vi "CreatePrivateEvents.vi"(8 "error in (no error)":errorcluster, 11 "Lockin.DAQ":refnum<class "Instrument.DAQ.lvclass">) -> (0 "error out":errorcluster, 3 "Lockin.DAQ out":refnum<class "Instrument.DAQ.lvclass">)   [LabVIEW 2019, in "Instrument.Lockin.lvlib" / "Instrument.DAQ.lvclass"]
doc: "---------------------------------------------------------------\nJKI State Machine Objects™\nhttp://jki.net/state-machine-objects/\nCopyright (C) 2005-2015, JKI <info@jki.net>\nALL RIGHTS RESERVEDJKI State Machine Objects (SMO) 1.0.0.4\nJKI - JKI\nCopyright (c) 2015, JKI"
uses:
  Instrument.DAQ.lvclass
  Typedefs/PrivateEvents--DAQ.setAOconfig.ctl
  Typedefs/DAQ.Config.AO--Cluster--Array.ctl
  Typedefs/DAQ.Config.AO--Cluster.ctl
  Typedefs/DAQ.Config.AO.Range--enum.ctl
  Typedefs/DAQ.Type--enum.ctl
  Typedefs/PrivateEvents--DAQ.setAIconfig.ctl
  Typedefs/DAQ.Config.AI--Cluster--Array.ctl
  Typedefs/DAQ.Config.AI--Cluster.ctl
  Typedefs/DAQ.Config.AI.Coupling--enum.ctl
  Typedefs/DAQ.Config.AI.Range--enum.ctl
  Typedefs/Simulation Mode--enum.ctl
  Typedefs/PrivateEvents--DAQ.setAO.ctl
  Typedefs/AO.Channel--Cluster--Array.ctl
  Typedefs/AO.Channel--Cluster.ctl
  Typedefs/AO.Channel.Function--Enum.ctl
  Typedefs/PrivateEvents--DAQ.setREF.ctl
  Typedefs/REF.Channel--Cluster--Array.ctl
  Typedefs/REF.Channel--Cluster.ctl
  Typedefs/PrivateEvents--DAQ.setSampling.ctl
  Typedefs/DAQ.Sampling--Cluster.ctl
  Typedefs/DAQ.Sampling.Sampling--Cluster.ctl
  Typedefs/DAQ.Sampling.Fs Mode--enum.ctl
  Typedefs/PrivateEvents--DAQ.setState.ctl
  Typedefs/Set State-enum.ctl
  Typedefs/PrivateEvents--DAQ.setInputGain.ctl
  Typedefs/PrivateEvents--DAQ.setSweep.ctl
  Typedefs/Sweep.Configuration--Cluster.ctl
  Typedefs/Sweep.Channel--Cluster--Array.ctl
  Typedefs/Sweep.Channel--Cluster.ctl
  Typedefs/Sweep.Pattern--Enum.ctl
  Typedefs/PrivateEvents--DAQ.measureOffset.ctl
  Typedefs/PrivateEvents--DAQ.zeroOffset.ctl
  Typedefs/PrivateEvents--DAQ.setPreFilter.ctl
  Typedefs/Configuration.Prefilter--Cluster.ctl
  Typedefs/PrivateEvents--DAQ.autoConfigureDAQ.ctl
  Typedefs/PrivateEvents--DAQ.setCalibration.ctl
  Typedefs/PrivateEvents--DAQ.setOutputGain.ctl
  Typedefs/PrivateEvents--DAQ.setAI.ctl
  Typedefs/AI.Channel--Cluster--Array.ctl
  Typedefs/AI.Channel--Cluster.ctl
  Typedefs/PrivateEvents--DAQ.zeroPhase.ctl
  Typedefs/PrivateEvents--DAQ.setAmplitudeLimit.ctl
  Typedefs/Configuration.AmplitudeLimit--Cluster.ctl
  Typedefs/PrivateEvents--DAQ.setLinkFrequencies.ctl
  Typedefs/Configuration.LinkFrequencies--Cluster.ctl
  Typedefs/PrivateEvents--DAQ.showUI.ctl
  Typedefs/PrivateEvents--DAQ.setInputOffset.ctl
  Instrument.DAQ.lvclass/Instrument.DAQ.ctl
  <vilib>/JKI/JKI SMO/SMO/SMO.lvclass
  Typedefs/Configuration.DCLimit--Cluster.ctl
  Typedefs/PrivateEvents--DAQ.setDCLimit.ctl
panel:
  # "For instructions on how to use the JKI State Machine Objects, examples and video tutorials, visit:\nhttp://jki.net/state-machine-objects/\n\nJKI State Machine Objects™\nhttp://jki.net/state-machine-objects/\nCopyright (C) 2005-2015, JKI <info@jki.net>\nALL RIGHTS RESERVED"
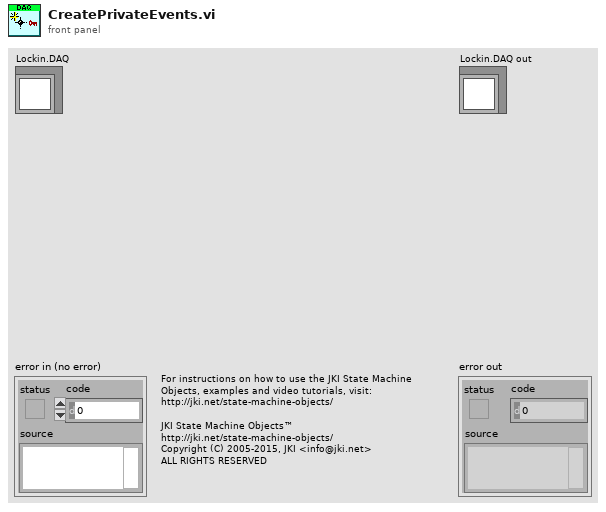
[diagram p1: front panel]
types:
  T1 = typedef "Instrument.Lockin.lvlib/Instrument.DAQ.lvclass/PrivateEvents--DAQ.setDCLimit.ctl" = cluster{"DC Limit":T2}
  T2 = typedef "Instrument.Lockin.lvlib/Instrument.DAQ.lvclass/Configuration.DCLimit--Cluster.ctl" = cluster{"Limit?":bool, "Limit (V)":dbl}
  T3 = typedef "Instrument.Lockin.lvlib/Instrument.DAQ.lvclass/PrivateEvents--DAQ.setInputOffset.ctl" = cluster{"Input Offset":dbl[]}
  T4 = typedef "Instrument.Lockin.lvlib/Instrument.DAQ.lvclass/PrivateEvents--DAQ.showUI.ctl" = bool
  T5 = typedef "Instrument.Lockin.lvlib/Instrument.DAQ.lvclass/PrivateEvents--DAQ.setLinkFrequencies.ctl" = cluster{"Link Frequencies":T6}
  T6 = typedef "Instrument.Lockin.lvlib/Instrument.DAQ.lvclass/Configuration.LinkFrequencies--Cluster.ctl" = cluster{"Link?":bool, "Frequency (Hz)":dbl}
  T7 = typedef "Instrument.Lockin.lvlib/Instrument.DAQ.lvclass/PrivateEvents--DAQ.setAmplitudeLimit.ctl" = cluster{"Amplitude Limit ":T8}
  T8 = typedef "Instrument.Lockin.lvlib/Instrument.DAQ.lvclass/Configuration.AmplitudeLimit--Cluster.ctl" = cluster{"Limit?":bool, "Limit (V)":dbl}
  T9 = typedef "Instrument.Lockin.lvlib/Instrument.DAQ.lvclass/PrivateEvents--DAQ.zeroPhase.ctl" = bool
  T10 = typedef "Instrument.Lockin.lvlib/Instrument.DAQ.lvclass/PrivateEvents--DAQ.setAI.ctl" = cluster{"AI Channels":T11}
  T11 = typedef "Instrument.Lockin.lvlib/Instrument.DAQ.lvclass/AI.Channel--Cluster--Array.ctl" = T12[]
  T12 = typedef "Instrument.Lockin.lvlib/Instrument.DAQ.lvclass/AI.Channel--Cluster.ctl" = cluster{"Enable?":bool, "Channel":i32, "References":i32[]}
  T13 = typedef "Instrument.Lockin.lvlib/Instrument.DAQ.lvclass/PrivateEvents--DAQ.setOutputGain.ctl" = cluster{"Output Gain":dbl[]}
  T14 = typedef "Instrument.Lockin.lvlib/Instrument.DAQ.lvclass/PrivateEvents--DAQ.setCalibration.ctl" = enum16{"Check", "Calibrate"}
  T15 = typedef "Instrument.Lockin.lvlib/Instrument.DAQ.lvclass/PrivateEvents--DAQ.autoConfigureDAQ.ctl" = bool
  T16 = typedef "Instrument.Lockin.lvlib/Instrument.DAQ.lvclass/PrivateEvents--DAQ.setPreFilter.ctl" = cluster{"PreFilter":T17}
  T17 = typedef "Instrument.Lockin.lvlib/Instrument.DAQ.lvclass/Configuration.Prefilter--Cluster.ctl" = cluster{"60 Hz":bool, "Low Pass":bool, "Low Pass Cutoff (Hz)":dbl}
  T18 = typedef "Instrument.Lockin.lvlib/Instrument.DAQ.lvclass/PrivateEvents--DAQ.zeroOffset.ctl" = bool
  T19 = typedef "Instrument.Lockin.lvlib/Instrument.DAQ.lvclass/PrivateEvents--DAQ.measureOffset.ctl" = bool
  T20 = typedef "Instrument.Lockin.lvlib/Instrument.DAQ.lvclass/PrivateEvents--DAQ.setSweep.ctl" = cluster{"setSweep":T21}
  T21 = typedef "Instrument.Lockin.lvlib/Instrument.DAQ.lvclass/Sweep.Configuration--Cluster.ctl" = cluster{"Sweep Time (s)":dbl, "Initial Wait (s)":dbl, "Return to Start":bool, "Channels":T22}
  T22 = typedef "Instrument.Lockin.lvlib/Instrument.DAQ.lvclass/Sweep.Channel--Cluster--Array.ctl" = T23[]
  T23 = typedef "Instrument.Lockin.lvlib/Instrument.DAQ.lvclass/Sweep.Channel--Cluster.ctl" = cluster{"Enable?":bool, "Channel":u16, "Start":dbl, "End":dbl, "Pattern":T24, "Table":dbl[]}
  T24 = typedef "Instrument.Lockin.lvlib/Instrument.DAQ.lvclass/Sweep.Pattern--Enum.ctl" = enum16{"Ramp /", "Ramp /\\", "Smooth Ramp _/", "Smooth Ramp _/\\_", "Table"}
  T25 = typedef "Instrument.Lockin.lvlib/Instrument.DAQ.lvclass/PrivateEvents--DAQ.setInputGain.ctl" = cluster{"Input Gain":dbl[]}
  T26 = typedef "Instrument.Lockin.lvlib/Instrument.DAQ.lvclass/PrivateEvents--DAQ.setState.ctl" = cluster{"setState":T27}
  T27 = typedef "Instrument.Lockin.lvlib/Instrument.DAQ.lvclass/Set State-enum.ctl" = enum16{"start", "stop", "reset", "start sweep", "stop sweep"}
  T28 = typedef "Instrument.Lockin.lvlib/Instrument.DAQ.lvclass/PrivateEvents--DAQ.setSampling.ctl" = cluster{"Sampling":T29}
  T29 = typedef "Instrument.Lockin.lvlib/Instrument.DAQ.lvclass/DAQ.Sampling--Cluster.ctl" = cluster{"Sampling":T30, "sample mode":i32, "Fs Mode":T31, "Fs Multiplier":dbl, "Refresh Rate (Hz)":dbl, "Decimation.PreDSP":i32, "Decimation.PostDSP":i32, "Fs.Output":dbl}
  T30 = typedef "Instrument.Lockin.lvlib/Instrument.DAQ.lvclass/DAQ.Sampling.Sampling--Cluster.ctl" = cluster{"Fs":dbl, "#s":i32}
  T31 = typedef "Instrument.Lockin.lvlib/Instrument.DAQ.lvclass/DAQ.Sampling.Fs Mode--enum.ctl" = enum16{"Manual", "Auto Fs", "Max Fs"}
  T32 = typedef "Instrument.Lockin.lvlib/Instrument.DAQ.lvclass/PrivateEvents--DAQ.setREF.ctl" = cluster{"REF Channels":T33}
  T33 = typedef "Instrument.Lockin.lvlib/Instrument.DAQ.lvclass/REF.Channel--Cluster--Array.ctl" = T34[]
  T34 = typedef "Instrument.Lockin.lvlib/Instrument.DAQ.lvclass/REF.Channel--Cluster.ctl" = cluster{"Enable?":bool, "Channel":i32, "Frequency":dbl, "Phase":dbl, "TC":dbl, "Roll-Off":i32}
  T35 = typedef "Instrument.Lockin.lvlib/Instrument.DAQ.lvclass/PrivateEvents--DAQ.setAO.ctl" = cluster{"AO Channels":T36}
  T36 = typedef "Instrument.Lockin.lvlib/Instrument.DAQ.lvclass/AO.Channel--Cluster--Array.ctl" = T37[]
  T37 = typedef "Instrument.Lockin.lvlib/Instrument.DAQ.lvclass/AO.Channel--Cluster.ctl" = cluster{"Enable?":bool, "Channel":i32, "Amplitude":dbl, "Offset":dbl, "Frequency":dbl, "Phase":dbl, "Function":T38, "Sweeping?":bool}
  T38 = typedef "Instrument.Lockin.lvlib/Instrument.DAQ.lvclass/AO.Channel.Function--Enum.ctl" = enum16{"Sine", "Triangle", "Square"}
  T39 = typedef "Instrument.Lockin.lvlib/Instrument.DAQ.lvclass/PrivateEvents--DAQ.setAIconfig.ctl" = cluster{"AI Configuration":T40, "Simulation mode":T45}
  T40 = typedef "Instrument.Lockin.lvlib/Instrument.DAQ.lvclass/DAQ.Config.AI--Cluster--Array.ctl" = T41[]
  T41 = typedef "Instrument.Lockin.lvlib/Instrument.DAQ.lvclass/DAQ.Config.AI--Cluster.ctl" = cluster{"Channels":tag, "Coupling":T42, "Range":T43, "input terminal configuration":i32, "Type":T44}
  T42 = typedef "Instrument.Lockin.lvlib/Instrument.DAQ.lvclass/DAQ.Config.AI.Coupling--enum.ctl" = u16
  T43 = typedef "Instrument.Lockin.lvlib/Instrument.DAQ.lvclass/DAQ.Config.AI.Range--enum.ctl" = enum16{"±0.316", "±1.00", "±3.16", "±10.0", "±31.6", "±42.4"}
  T44 = typedef "Instrument.Lockin.lvlib/Instrument.DAQ.lvclass/DAQ.Type--enum.ctl" = enum16{"None", "USB-4431", "PXI-446x"}
  T45 = typedef "Instrument.Lockin.lvlib/Instrument.DAQ.lvclass/Simulation Mode--enum.ctl" = enum16{"AI = HW simulated", "AI = noise*AO", "AI = waveguide"}
  T46 = typedef "Instrument.Lockin.lvlib/Instrument.DAQ.lvclass/PrivateEvents--DAQ.setAOconfig.ctl" = cluster{"AO Configuration":T47}
  T47 = typedef "Instrument.Lockin.lvlib/Instrument.DAQ.lvclass/DAQ.Config.AO--Cluster--Array.ctl" = T48[]
  T48 = typedef "Instrument.Lockin.lvlib/Instrument.DAQ.lvclass/DAQ.Config.AO--Cluster.ctl" = cluster{"Channels":tag, "Range":T49, "output terminal configuration":i32, "Type":T44}
  T49 = typedef "Instrument.Lockin.lvlib/Instrument.DAQ.lvclass/DAQ.Config.AO.Range--enum.ctl" = enum16{"±0.1", "±1.0", "±10.0"}
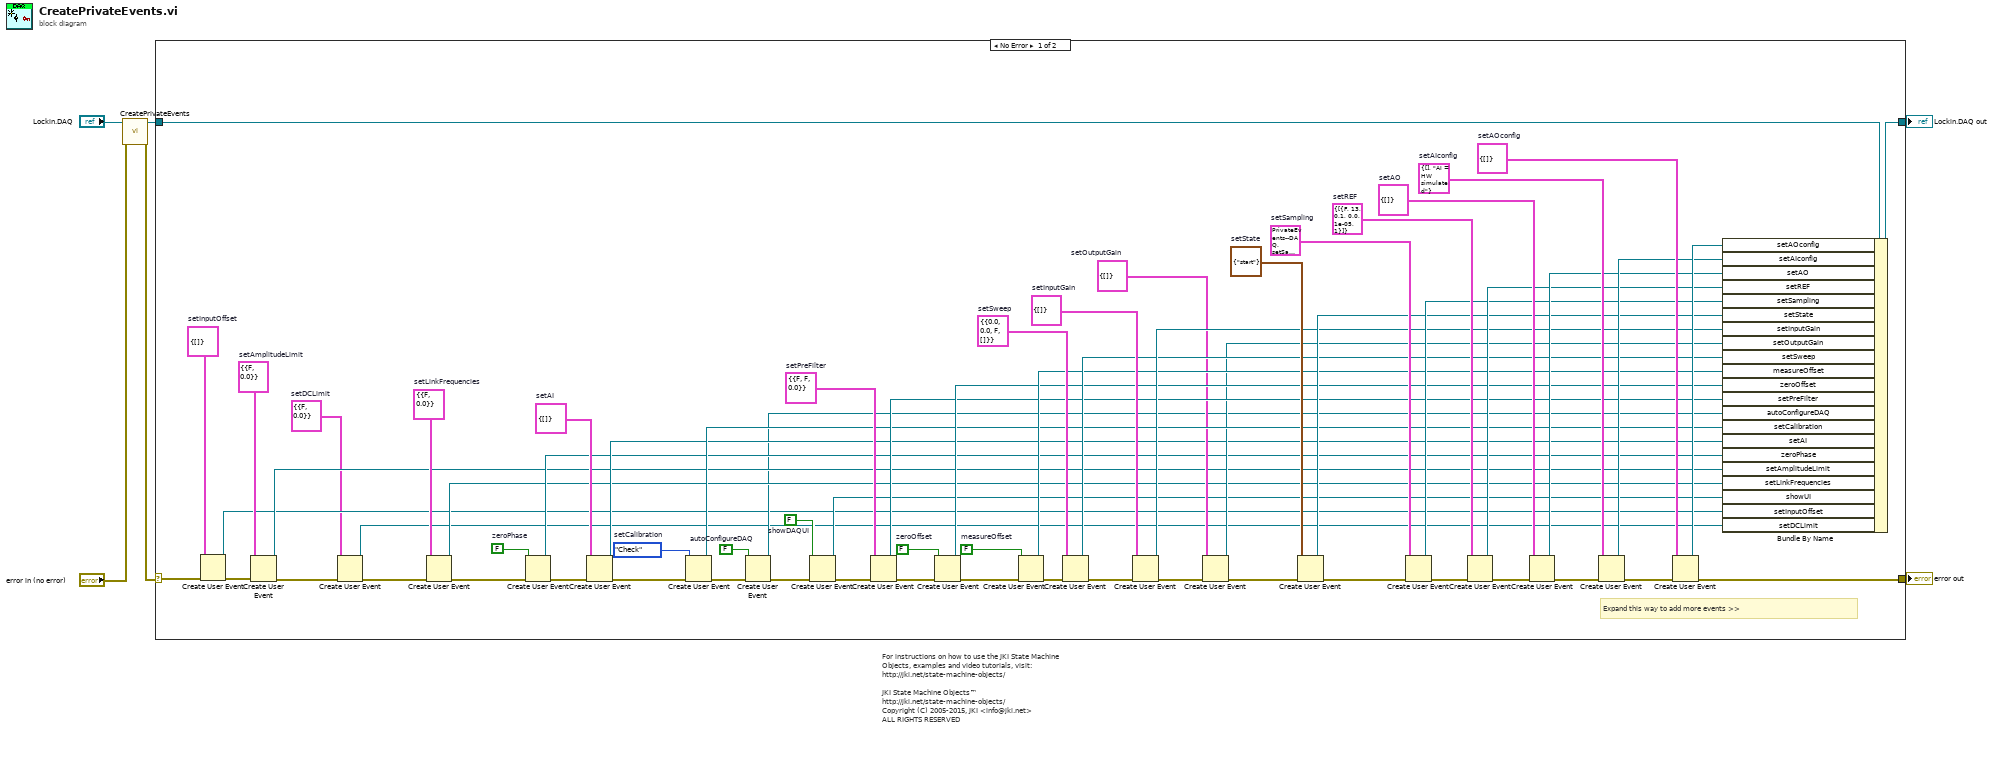
[diagram p0: block diagram]
diagram:
  # "For instructions on how to use the JKI State Machine Objects, examples and video tutorials, visit:\nhttp://jki.net/state-machine-objects/\n\nJKI State Machine Objects™\nhttp://jki.net/state-machine-objects/\nCopyright (C) 2005-2015, JKI <info@jki.net>\nALL RIGHTS RESERVED"
  n1 = call-parent "CreatePrivateEvents.vi"("error in (no error)"="error in (no error)", "SMO"="Lockin.DAQ") -> ("error out"=w1:errorcluster, "SMO out"=w3:refnum<class "Instrument.DAQ.lvclass">)  [unwired: 8 in]
  n2 = case shown="No Error" w1 {
    selector: w1 -> [w13 w74]
    tunnel: [w70 w74] -> w5
    tunnel: [w71 w73] -> w6
    tunnel: w3 -> [w72 w73]
    frame No Error {
      w10 = T1 {"DC Limit"={"Limit?"=FALSE, "Limit (V)"=0.0}}  # setDCLimit
      w14 = T3 {"Input Offset"=[]}  # setInputOffset
      w18 = T4 FALSE  # showDAQUI
      w22 = T5 {"Link Frequencies"={"Link?"=FALSE, "Frequency (Hz)"=0.0}}  # setLinkFrequencies
      w23 = T7 {"Amplitude Limit "={"Limit?"=FALSE, "Limit (V)"=0.0}}  # setAmplitudeLimit
      w26 = T9 FALSE  # zeroPhase
      w29 = T10 {"AI Channels"=[]}  # setAI
      w32 = T13 {"Output Gain"=[]}  # setOutputGain
      w36 = PrivateEvents--DAQ.setCalibration."Check"  # setCalibration
      w38 = T15 FALSE  # autoConfigureDAQ
      w40 = T16 {"PreFilter"={"60 Hz"=FALSE, "Low Pass"=FALSE, "Low Pass Cutoff (Hz)"=0.0}}  # setPreFilter
      w43 = T18 FALSE  # zeroOffset
      w46 = T19 FALSE  # measureOffset
      w49 = T20 {"setSweep"={"Sweep Time (s)"=0.0, "Initial Wait (s)"=0.0, "Return to Start"=FALSE, "Channels"=[]}}  # setSweep
      w52 = T25 {"Input Gain"=[]}  # setInputGain
      w54 = T26 {"setState"=enum."start"}  # setState
      w57 = T28 {"Sampling"={"Sampling"={"Fs"=10178.0, "#s"=100}, "sample mode"=15753, "Fs Mode"=enum."Max Fs", "Fs Multiplier"=1.0, "Refresh Rate (Hz)"=10.0, "Decimation.PreDSP"=1, "Decimation.PostDSP"=1, "Fs.Output"=204789.0}}  # setSampling
      w60 = T32 {"REF Channels"=[{"Enable?"=FALSE, "Channel"=13, "Frequency"=0.1, "Phase"=0.0, "TC"=1e-05, "Roll-Off"=1}]}  # setREF
      w63 = T35 {"AO Channels"=[]}  # setAO
      w66 = T39 {"AI Configuration"=[], "Simulation mode"=enum."AI = HW simulated"}  # setAIconfig
      w69 = T46 {"AO Configuration"=[]}  # setAOconfig
      # "Expand this way to add more events >>"
      n3 = Create User Event(user event datatype=w14, error in=w13) -> (user event=w11:refnum<user-event>, error out=w12:errorcluster)
      n4 = Create User Event(user event datatype=w23, error in=w12) -> (user event=w21:refnum<user-event>, error out=w9:errorcluster)
      n5 = Create User Event(user event datatype=w10, error in=w9) -> (user event=w7:refnum<user-event>, error out=w8:errorcluster)
      n6 = Create User Event(user event datatype=w22, error in=w8) -> (user event=w20:refnum<user-event>, error out=w24:errorcluster)
      n7 = Create User Event(user event datatype=w26, error in=w24) -> (user event=w25:refnum<user-event>, error out=w27:errorcluster)
      n8 = Create User Event(user event datatype=w29, error in=w27) -> (user event=w28:refnum<user-event>, error out=w30:errorcluster)
      n9 = Create User Event(user event datatype=w36, error in=w30) -> (user event=w35:refnum<user-event>, error out=w37:errorcluster)
      n10 = Create User Event(user event datatype=w38, error in=w37) -> (user event=w19:refnum<user-event>, error out=w17:errorcluster)
      n11 = Create User Event(user event datatype=w18, error in=w17) -> (user event=w16:refnum<user-event>, error out=w15:errorcluster)
      n12 = Create User Event(user event datatype=w40, error in=w15) -> (user event=w39:refnum<user-event>, error out=w41:errorcluster)
      n13 = Create User Event(user event datatype=w43, error in=w41) -> (user event=w42:refnum<user-event>, error out=w44:errorcluster)
      n14 = Create User Event(user event datatype=w46, error in=w44) -> (user event=w45:refnum<user-event>, error out=w47:errorcluster)
      n15 = Create User Event(user event datatype=w49, error in=w47) -> (user event=w48:refnum<user-event>, error out=w50:errorcluster)
      n16 = Create User Event(user event datatype=w52, error in=w50) -> (user event=w51:refnum<user-event>, error out=w34:errorcluster)
      n17 = Create User Event(user event datatype=w32, error in=w34) -> (user event=w31:refnum<user-event>, error out=w33:errorcluster)
      n18 = Create User Event(user event datatype=w54, error in=w33) -> (user event=w53:refnum<user-event>, error out=w55:errorcluster)
      n19 = Create User Event(user event datatype=w57, error in=w55) -> (user event=w56:refnum<user-event>, error out=w58:errorcluster)
      n20 = Create User Event(user event datatype=w60, error in=w58) -> (user event=w59:refnum<user-event>, error out=w61:errorcluster)
      n21 = Create User Event(user event datatype=w63, error in=w61) -> (user event=w62:refnum<user-event>, error out=w64:errorcluster)
      n22 = Create User Event(user event datatype=w66, error in=w64) -> (user event=w65:refnum<user-event>, error out=w67:errorcluster)
      n23 = Create User Event(user event datatype=w69, error in=w67) -> (user event=w68:refnum<user-event>, error out=w70:errorcluster)
      n24 = Bundle By Name(cluster=w72, "setAOconfig"=w68, "setAIconfig"=w65, "setAO"=w62, "setREF"=w59, "setSampling"=w56, "setState"=w53, "setInputGain"=w51, "setOutputGain"=w31, "setSweep"=w48, "measureOffset"=w45, "zeroOffset"=w42, "setPreFilter"=w39, "autoConfigureDAQ"=w19, "setCalibration"=w35, "setAI"=w28, "zeroPhase"=w25, "setAmplitudeLimit"=w21, "setLinkFrequencies"=w20, "showUI"=w16, "setInputOffset"=w11, "setDCLimit"=w7) -> (w71:refnum<class "Instrument.DAQ.lvclass">)
    }
    frame Error {
    }
  }
  "error out" <- w5
  "Lockin.DAQ out" <- w6
